vi "DC40_Example.vi"() -> ()   [LabVIEW 2023]
panel:
  out "LED Current Limit":dbl
  in  "LED Current [A]":dbl(slide) scale=0.0..1.2
  in  "?":bool
  in  "Enable LED Output":bool=TRUE caption="Enable LED Output (On)"
  out "LED Wavelength":dbl
  out "LED Serial Number":string
  out "LED Name":string
  out "LED Forward Voltage":dbl
  # "DC40 Example"
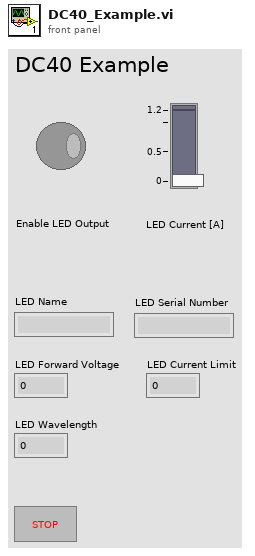
[diagram p1: front panel]
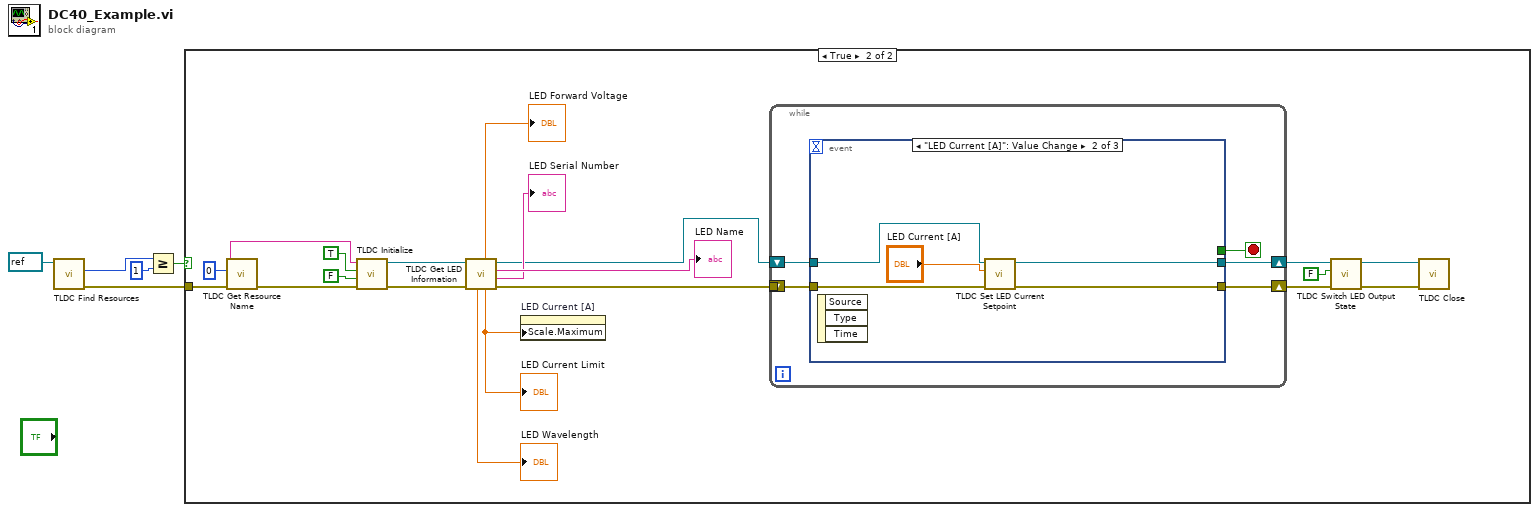
[diagram p0: block diagram]
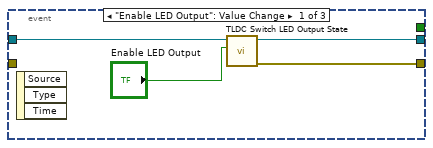
[diagram p3: hidden frame]
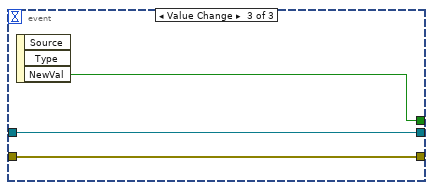
[diagram p4: hidden frame]
diagram:
  n1 = call "TLDC Find Resources.vi"("instrument handle"=refnum<visa-resource-name> refnum) -> ("error out"=w1:errorcluster, "Resource Count"=w3:u32)  [unwired: 8 in, 1 out]
  n2 = Greater Or Equal?(x=w3, y=u32 1) -> (x >= y?=w4:bool)
  n3 = case shown="True" w4 {
    tunnel: w1 -> [_ w24]
    frame False {
    }
    frame True {
      n4 = call "TLDC Get Resource Name.vi"("error in (no error)"=w24, "Index (0)"=u32 0) -> ("error out"=w20:errorcluster, "Resource Name"=w23:string)  [unwired: 7 in, 1 out]
      n5 = call "TLDC Initialize.vi"("error in (no error)"=w20, "Reset Device (Yes)"=FALSE, "ID Query (Yes)"=TRUE, "resource name"=w23) -> ("error out"=w18:errorcluster, "instrument handle out"=w19:refnum<visa-resource-name>)  [unwired: 6 in]
      n6 = call "TLDC Get LED Information.vi"("error in (no error)"=w18, "instrument handle"=w19) -> ("error out"=w12:errorcluster, "LED Serial Number"=→"LED Serial Number":string, "LED Name"=→"LED Name":string, "instrument handle out"=w13:refnum<visa-resource-name>, "LED Current Limit"=w11:dbl, "LED Forward Voltage"=→"LED Forward Voltage":dbl, "LED Wavelength"=→"LED Wavelength":dbl)  [unwired: 3 in]
      "LED Current Limit" <- w11
      n7 = property on="LED Current [A]" class="Slide (strict)"("Scale.Maximum"=w11) -> ()  [unwired: 2 in, 2 out]
      n8 = while {
        shift-right: [w29] -> w10
        shift-left: w13 -> [w30]
        tunnel: w12 -> [w27]
        shift-right: [w28] -> w9
        shift-left: _ -> [_]
        stop <- w26 stop-if-true
        n9 = event shown="[1] \"LED Current [A]\": Value Change" {
          selector: _ -> [_ _ _]
          dyn-events: _ -> [_ _ _]
          timeout: _ -> [_ _ _]
          tunnel: w30 -> [w34 w39 w42]
          tunnel: [w32 w38 w42] -> w29
          tunnel: [w31 w36 w41] -> w28
          tunnel: w27 -> [_ w37 w41]
          tunnel: [_ _ w40] -> w26
          event "Enable LED Output": Value Change {
            n10 = event-data() -> ()  [unwired: 1 in, 3 out]
            n11 = call "TLDC Switch LED Output State.vi"("Enable LED Output (On)"="Enable LED Output", "instrument handle"=w34) -> ("error out"=w31:errorcluster, "instrument handle out"=w32:refnum<visa-resource-name>)  [unwired: 8 in]
          }
          event "LED Current [A]": Value Change {
            n12 = event-data() -> ()  [unwired: 1 in, 3 out]
            n13 = call "TLDC Set LED Current Setpoint.vi"("error in (no error)"=w37, "LED Current Setpoint (0.0)"="LED Current [A]", "instrument handle"=w39) -> ("error out"=w36:errorcluster, "instrument handle out"=w38:refnum<visa-resource-name>)  [unwired: 7 in]
          }
          event Value Change {
            n14 = event-data() -> ("NewVal"=w40:bool)  [unwired: 1 in, 2 out]
          }
        }
      }
      n15 = call "TLDC Switch LED Output State.vi"("error in (no error)"=w9, "Enable LED Output (On)"=FALSE, "instrument handle"=w10) -> ("error out"=w7:errorcluster, "instrument handle out"=w8:refnum<visa-resource-name>)  [unwired: 7 in]
      n16 = call "TLDC Close.vi"("error in (no error)"=w7, "instrument handle"=w8) -> ()  [unwired: 9 in, 1 out]
    }
  }
